vi "Keithley2400 Set Range-Compliance.vi"(8 "error in (no error)":errorcluster, 9 "Voltage range (V)":dbl=20.0, 10 "Compliance (A)":dbl=0.001, 11 "VISA Refnum in":refnum<visa-resource-name>) -> (0 "error out":errorcluster, 3 "VISA Refnum out":refnum<visa-resource-name>)   [LabVIEW 2018]
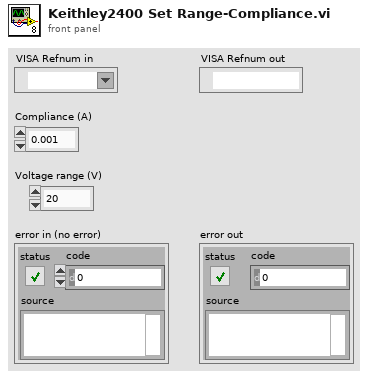
[diagram p1: front panel]
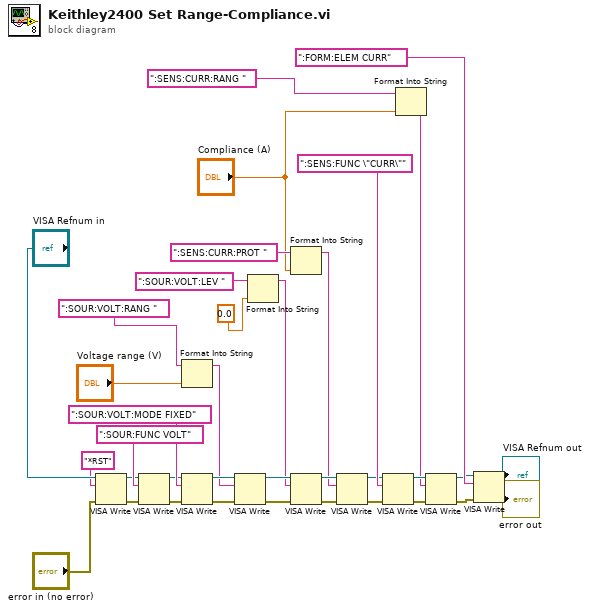
[diagram p0: block diagram]
diagram:
  n1 = VISA Write(VISA resource name="VISA Refnum in", write buffer="*RST", error in (no error)="error in (no error)") -> (VISA resource name out=w26:refnum<visa-resource-name>, error out=w18:errorcluster)  [unwired: 1 out]
  n2 = VISA Write(VISA resource name=w26, write buffer=":SOUR:FUNC VOLT", error in (no error)=w18) -> (VISA resource name out=w25:refnum<visa-resource-name>, error out=w17:errorcluster)  [unwired: 1 out]
  n3 = Format Into String(initial string=":SOUR:VOLT:RANG " ("write buffer"), "Voltage range (V)") -> (resulting string=w7:string)  [unwired: 2 in, 1 out]
  n4 = VISA Write(VISA resource name=w25, write buffer=":SOUR:VOLT:MODE FIXED", error in (no error)=w17) -> (VISA resource name out=w24:refnum<visa-resource-name>, error out=w16:errorcluster)  [unwired: 1 out]
  n5 = VISA Write(VISA resource name=w24, write buffer=w7, error in (no error)=w16) -> (VISA resource name out=w23:refnum<visa-resource-name>, error out=w15:errorcluster)  [unwired: 1 out]
  n6 = Format Into String(initial string=":SOUR:VOLT:LEV " ("write buffer"), 0.0 ("input 1")) -> (resulting string=w9:string)  [unwired: 2 in, 1 out]
  n7 = Format Into String(initial string=":SENS:CURR:PROT " ("write buffer"), "Compliance (A)") -> (resulting string=w5:string)  [unwired: 2 in, 1 out]
  n8 = VISA Write(VISA resource name=w23, write buffer=w9, error in (no error)=w15) -> (VISA resource name out=w22:refnum<visa-resource-name>, error out=w14:errorcluster)  [unwired: 1 out]
  n9 = VISA Write(VISA resource name=w22, write buffer=w5, error in (no error)=w14) -> (VISA resource name out=w21:refnum<visa-resource-name>, error out=w13:errorcluster)  [unwired: 1 out]
  n10 = VISA Write(VISA resource name=w21, write buffer=":SENS:FUNC \"CURR\"", error in (no error)=w13) -> (VISA resource name out=w20:refnum<visa-resource-name>, error out=w12:errorcluster)  [unwired: 1 out]
  n11 = Format Into String(initial string=":SENS:CURR:RANG " ("write buffer"), "Compliance (A)") -> (resulting string=w2:string)  [unwired: 2 in, 1 out]
  n12 = VISA Write(VISA resource name=w20, write buffer=w2, error in (no error)=w12) -> (VISA resource name out=w19:refnum<visa-resource-name>, error out=w11:errorcluster)  [unwired: 1 out]
  n13 = VISA Write(VISA resource name=w19, write buffer=":FORM:ELEM CURR", error in (no error)=w11) -> (VISA resource name out=→"VISA Refnum out":refnum<visa-resource-name>, error out=→"error out":errorcluster)  [unwired: 1 out]
